vi "Climb Sequence.vi"   [LabVIEW 2012]
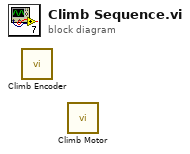
[diagram p0: block diagram]
diagram:
  n1 = call "Climb Encoder.vi"() -> ()  [unwired: 12 in]
  n2 = call "Climb Motor.vi"() -> ()  [unwired: 12 in]
